vi "Replacer(X...)to(0...)1.vi"(2 "[IN] Starting index":i32, 3 "[IN] Array":dbl[](array[numeric])) -> (0 "Finish index":i32, 1 "Replaced array":dbl[](array[numeric]))   [LabVIEW 2017]
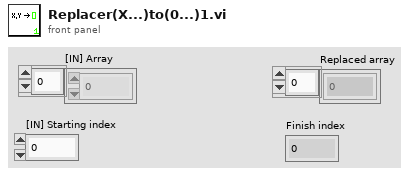
[diagram p1: front panel]
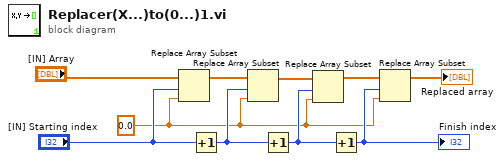
[diagram p0: block diagram]
diagram:
  w2 = 0.0 ("new element/subarray")
  n1 = Replace Array Subset(array="[IN] Array", new element=w2, index="[IN] Starting index") -> (w9:dbl[])
  n2 = Increment(x="[IN] Starting index") -> (x+1=w6:i32)
  n3 = Replace Array Subset(array=w9, new element=w2, index=w6) -> (w7:dbl[])
  n4 = Increment(x=w6) -> (x+1=w4:i32)
  n5 = Replace Array Subset(array=w7, new element=w2, index=w4) -> (w5:dbl[])
  n6 = Increment(x=w4) -> (x+1=w3:i32)
  "Finish index" <- w3
  n7 = Replace Array Subset(array=w5, new element=w2, index=w3) -> (→"Replaced array":dbl[])
